vi "Common.vi"(8 "error in (no error)":errorcluster, 9 "Action":T1=enum."TemplatesFolderName") -> (0 "error out":errorcluster, 1 "Output":string)   [LabVIEW 2014, in "CD model script.lvlib"]
doc: "Contains all constants, which are not part of specific part of the wizard."
uses:
  CD model script.lvlib
  Constants TypDef/Common.ctl
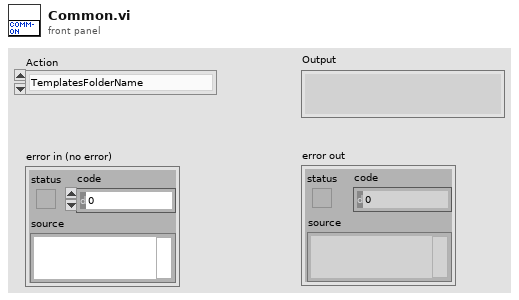
[diagram p1: front panel]
types:
  T1 = typedef "CD model script.lvlib/Common.ctl" = enum16{"ProjectName", "TemplatesFolderName", "ProjectTemplatePathAndName", "ReadmeTemplatePathAndName", "TimingAndSyncFolderName", "CustomDeviceFolderName"}
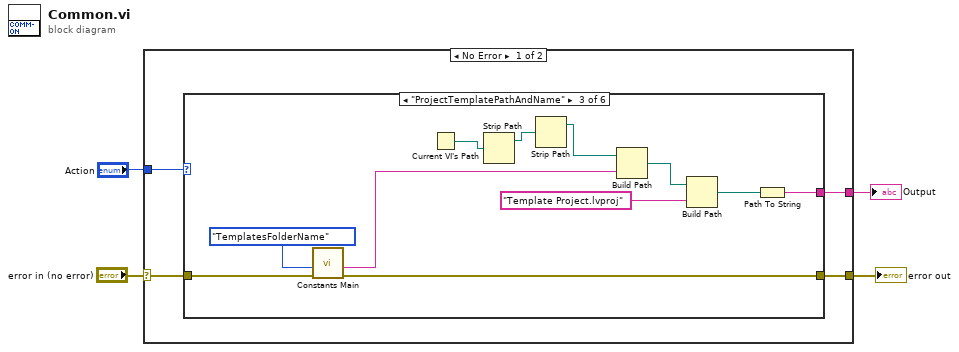
[diagram p0: block diagram]
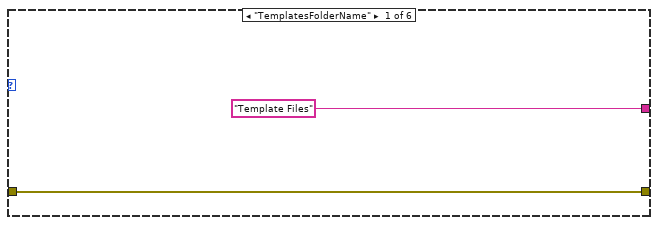
[diagram p2: hidden frame]
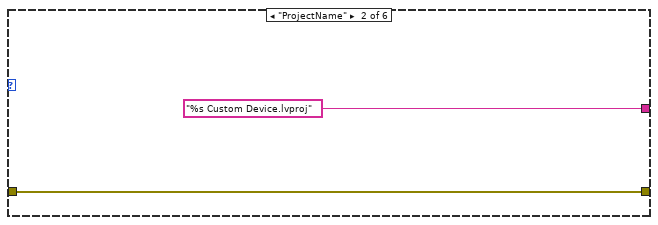
[diagram p3: hidden frame]
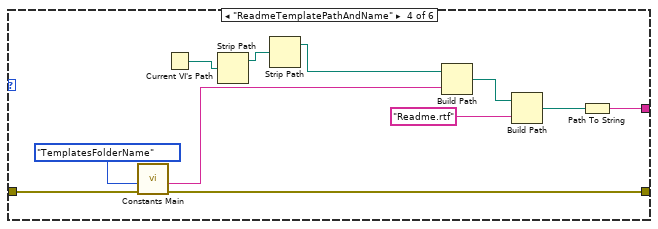
[diagram p4: hidden frame]
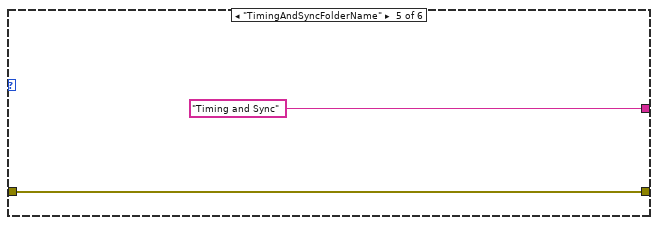
[diagram p5: hidden frame]
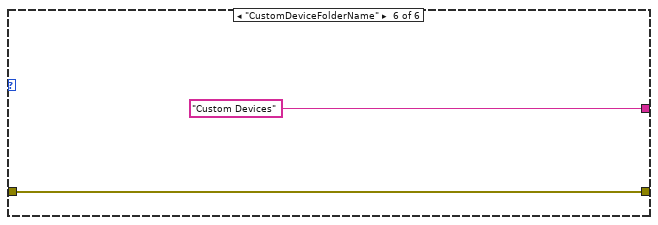
[diagram p6: hidden frame]
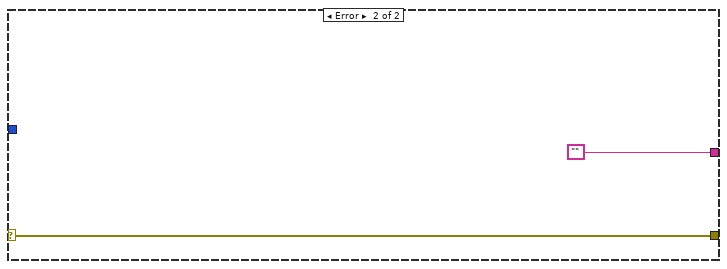
[diagram p7: hidden frame]
diagram:
  n1 = case shown="No Error" "error in (no error)" {
    selector: "error in (no error)" -> [w5 w40]
    tunnel: [w6 w40] -> w3
    tunnel: [w7 ""] -> w2
    tunnel: "Action" -> [w8 _]
    frame No Error {
      n2 = case shown="\"ProjectTemplatePathAndName\"" w8 {
        tunnel: ["Template Files" "%s Custom Device.lvproj" w16 w27 "Timing and Sync" "Custom Devices"] -> w7
        tunnel: [w9 w11 w17 w28 w35 w37] -> w6
        tunnel: w5 -> [w9 w11 w18 w29 w35 w37]
        frame "TemplatesFolderName" {
        }
        frame "ProjectName" {
        }
        frame "ProjectTemplatePathAndName" {
          n3 = call-poly "Constants Main.vi"("error in (no error)"=w18, "Action"=Common."TemplatesFolderName") -> ("error out"=w17:errorcluster, "Output"=w23:string)  [unwired: 8 in]
          n4 = Current VI's Path() -> (path=w15:path)
          n5 = Strip Path(path=w15) -> (stripped path=w14:path)  [unwired: 1 out]
          n6 = Strip Path(path=w14) -> (stripped path=w13:path)  [unwired: 1 out]
          n7 = Build Path(base path=w13, name or relative path=w23) -> (appended path=w22:path)
          n8 = Build Path(base path=w22, name or relative path="Template Project.lvproj") -> (appended path=w20:path)
          n9 = Path To String(path=w20) -> (string=w16:string)
        }
        frame "ReadmeTemplatePathAndName" {
          n10 = call-poly "Constants Main.vi"("error in (no error)"=w29, "Action"=Common."TemplatesFolderName") -> ("error out"=w28:errorcluster, "Output"=w34:string)  [unwired: 8 in]
          n11 = Current VI's Path() -> (path=w26:path)
          n12 = Strip Path(path=w26) -> (stripped path=w25:path)  [unwired: 1 out]
          n13 = Strip Path(path=w25) -> (stripped path=w24:path)  [unwired: 1 out]
          n14 = Build Path(base path=w24, name or relative path=w34) -> (appended path=w33:path)
          n15 = Build Path(base path=w33, name or relative path="Readme.rtf") -> (appended path=w31:path)
          n16 = Path To String(path=w31) -> (string=w27:string)
        }
        frame "TimingAndSyncFolderName" {
        }
        frame "CustomDeviceFolderName" {
        }
      }
    }
    frame Error {
    }
  }
  "error out" <- w3
  "Output" <- w2
